vi "Pulse once on press.vi"(1 "duration of pulse":dbl, 3 "in":bool) -> (0 "pulse":bool)   [LabVIEW 2017]
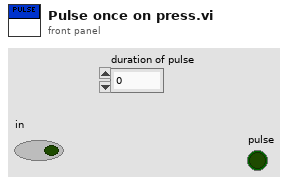
[diagram p1: front panel]
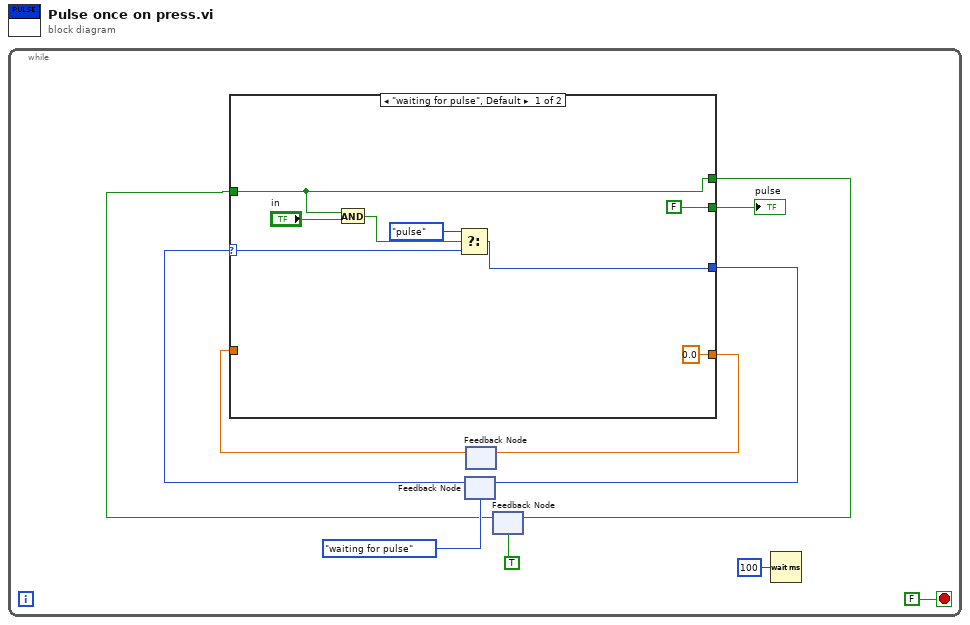
[diagram p0: block diagram]
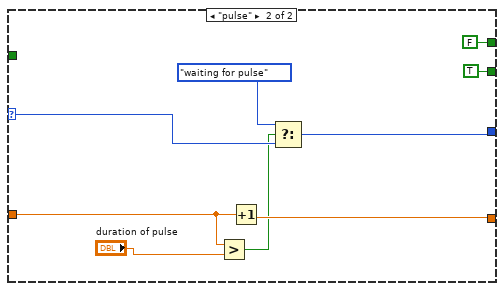
[diagram p2: hidden frame]
diagram:
  n1 = while {
    stop <- FALSE stop-if-true
    n2 = feedback #1(enum16{"waiting for pulse", "pulse"}."waiting for pulse") -> (w10:enum16{"waiting for pulse", "pulse"})
    n3 = feedback #2() -> (w6:dbl)  [unwired: 1 in]
    n4 = feedback #3(TRUE) -> (w4:bool)
    n5 = case shown="\"waiting for pulse\", Default" w10 {
      selector: w10 -> [w19 w26]
      tunnel: [w18 w27] -> w11
      tunnel: [FALSE TRUE] -> w8
      tunnel: w6 -> [_ w23]
      tunnel: [0.0 w24] -> w7
      tunnel: [w13 FALSE] -> w5
      tunnel: w4 -> [w13 _]
      frame "waiting for pulse", Default {
        n6 = And(x=w13, y="in") -> (x .and. y?=w15:bool)
        n7 = Select(t=enum16{"waiting for pulse", "pulse"}."pulse", s=w15, f=w19) -> (s? t:f=w18:enum16{"waiting for pulse", "pulse"})
      }
      frame "pulse" {
        n8 = Greater?(x=w23, y="duration of pulse") -> (0:w21:bool)
        n9 = Increment(x=w23) -> (x+1=w24:dbl)
        n10 = Select(t=enum16{"waiting for pulse", "pulse"}."waiting for pulse", s=w21, f=w26) -> (s? t:f=w27:enum16{"waiting for pulse", "pulse"})
      }
    }
    "pulse" <- w8
    n11 = feedback-in #1(w11) -> ()
    n12 = feedback-in #2(w7) -> ()
    n13 = feedback-in #3(w5) -> ()
    n14 = Wait (ms)(milliseconds to wait=u32 100) -> ()  [unwired: 1 out]
  }
